vi "SaveConfigFile.vi"(8 "error in (no error)":errorcluster, 11 "Microscope in":refnum<class "Microscope.lvclass">) -> (0 "error out":errorcluster, 3 "Microscope out":refnum<class "Microscope.lvclass">)   [LabVIEW 2020, in "Microscope.lvlib" / "Microscope.lvclass"]
uses:
  Microscope.lvclass
  Component/Device/Device/Device.lvclass
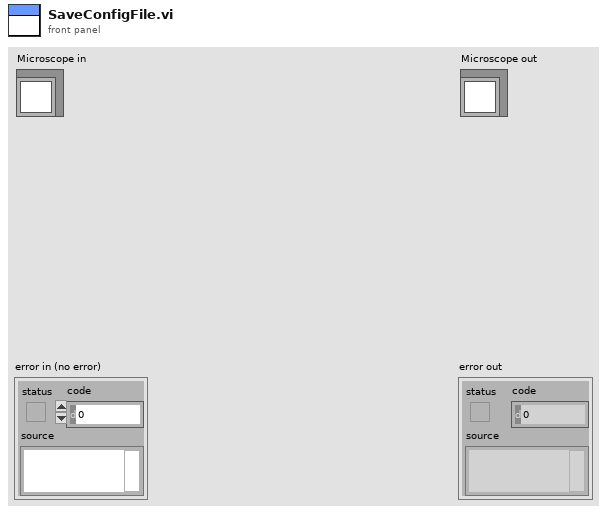
[diagram p1: front panel]
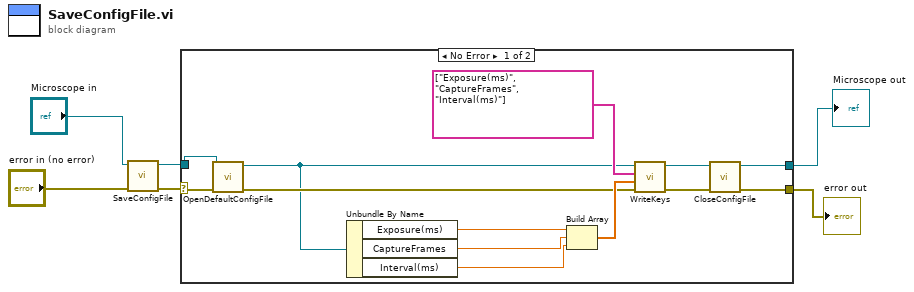
[diagram p0: block diagram]
diagram:
  n1 = call-parent "SaveConfigFile.vi"("error in (no error)"="error in (no error)", "Device in"="Microscope in") -> ("error out"=w4:errorcluster, "Device out"=w3:refnum<class "Microscope.lvclass">)  [unwired: 8 in]
  n2 = case shown="No Error" w4 {
    selector: w4 -> [w19 w20]
    tunnel: [w9 w20] -> w1
    tunnel: [w7 w21] -> w2
    tunnel: w3 -> [w11 w21]
    frame No Error {
      n3 = call-dynamic "OpenDefaultConfigFile.vi"("error in (no error)"=w19, "Device in"=w11) -> ("error out"=w12:errorcluster, "Device out"=w10:refnum<class "Microscope.lvclass">)  [unwired: 8 in]
      n4 = Unbundle By Name(w10) -> ("Exposure(ms)"=w16:dbl, "CaptureFrames"=w15:dbl, "Interval(ms)"=w14:dbl)
      n5 = Build Array(w16, w15, w14) -> (w13:dbl[])
      n6 = call-dynamic "WriteKeys.vi"("error in (no error)"=w12, "Value"=w13, "Keys"=string[] ["Exposure(ms)", "CaptureFrames", "Interval(ms)"], "Device in"=w10) -> ("error out"=w18:errorcluster, "Device out"=w8:refnum<class "Microscope.lvclass">)  [unwired: 6 in]
      n7 = call-dynamic "CloseConfigFile.vi"("error in (no error)"=w18, "GRMActor in"=w8) -> ("error out"=w9:errorcluster, "GRMActor out"=w7:refnum<class "Microscope.lvclass">)  [unwired: 8 in]
    }
    frame Error {
    }
  }
  "error out" <- w1
  "Microscope out" <- w2
